vi "Set User Interfaces.vi"(10 "User Interfaces":refnum<class "Component User Interfaces.lvclass">, 11 "Component in":refnum<class "Component.lvclass">) -> (3 "Component out":refnum<class "Component.lvclass">)   [LabVIEW 2019, in "DSF Core.lvlib" / "Component.lvclass"]
uses:
  Component.lvclass
  Component User Interface/Component User Interfaces.lvclass
  Component.lvclass/Component.ctl
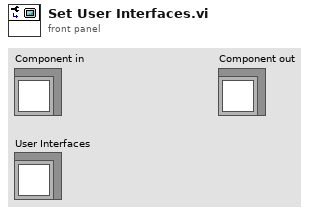
[diagram p1: front panel]
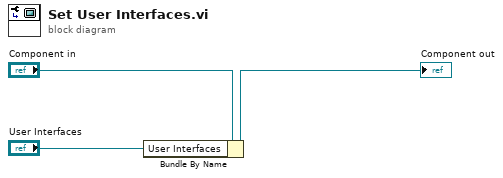
[diagram p0: block diagram]
diagram:
  n1 = Bundle By Name(cluster="Component in", "User Interfaces"="User Interfaces") -> (→"Component out":refnum<class "Component.lvclass">)
